vi "Set Button Complete.vi"(0 "Button in":refnum<class "Button.lvclass">, 1 "On Picture":picture, 2 "Disabled Picture":picture, 5 "Type":T1, 7 "State":T2, 9 "Off Picture":picture, 11 "error in (no error)":errorcluster, 12 "Hover Picture":picture, 13 "Button Size":i32) -> (4 "Button out":refnum<class "Button.lvclass">, 15 "error out":errorcluster)   [LabVIEW 2012, in "Button.lvclass"]
uses:
  Button.lvclass
  Type Defs/Button Status.ctl
  Type Defs/Button Type.ctl
  Button.lvclass/Button.ctl
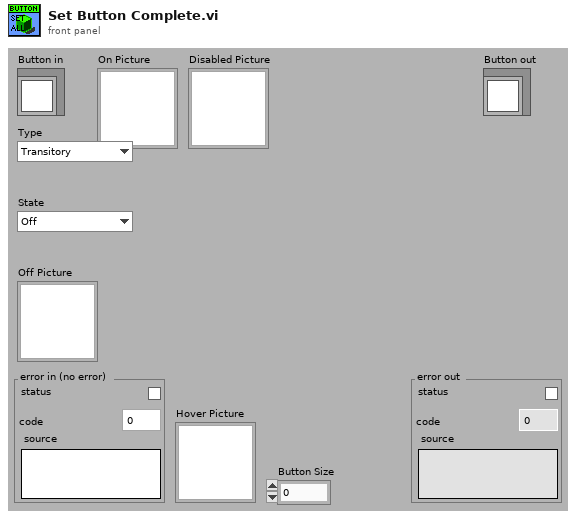
[diagram p1: front panel]
types:
  T1 = typedef "Button.lvclass/Button Type.ctl" = enum16{"Transitory", "Latching"}
  T2 = typedef "Button.lvclass/Button Status.ctl" = enum16{"Off", "Hover", "On", "Disabled"}
  T3 = typedef "imagedata.ctl" = cluster{"image type":i32, "image depth":i32, "image":u8[], "mask":u8[], "colors":u32[], "Rectangle":cluster{"left":i16, "top":i16, "right":i16, "bottom":i16}}
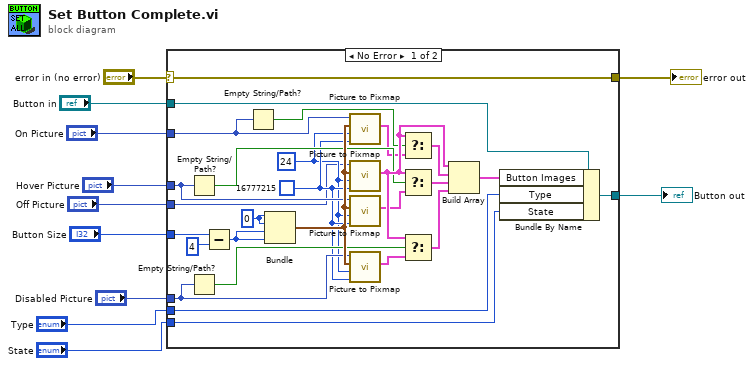
[diagram p0: block diagram]
diagram:
  n1 = case shown="No Error" "error in (no error)" {
    selector: "error in (no error)" -> [w12 w39]
    tunnel: "Button Size" -> [w36 _]
    tunnel: "Disabled Picture" -> [w22 _]
    tunnel: "Hover Picture" -> [w21 _]
    tunnel: "On Picture" -> [w18 _]
    tunnel: "Off Picture" -> [w17 _]
    tunnel: "State" -> [w16 _]
    tunnel: "Type" -> [w15 _]
    tunnel: [w14 w40] -> w4
    tunnel: "Button in" -> [w13 w40]
    tunnel: [w12 w39] -> w1
    frame No Error {
      w34 = 0
      w20 = u32 16777215 ("Background Color")
      w19 = 24 ("depth")
      n2 = Empty String/Path?(string/path=w21) -> (empty?=w25:bool)
      n3 = Empty String/Path?(string/path=w22) -> (empty?=w28:bool)
      n4 = Subtract(x=w36, y=4 ("x")) -> (x-y=w35:i32)
      n5 = Empty String/Path?(string/path=w18) -> (empty?=w23:bool)
      n6 = Bundle(w34, w34, w35, w35) -> (w33:cluster{i32, i32, i32, i32})  [unwired: 1 out]
      n7 = call <vilib>:"Picture to Pixmap.vi"("Background Color"=w20, "depth"=w19, "rect"=w33, "picture"=w18) -> ("image data"=w24:T3)  [unwired: 7 out]
      n8 = call <vilib>:"Picture to Pixmap.vi"("Background Color"=w20, "depth"=w19, "rect"=w33, "picture"=w17) -> ("image data"=w29:T3)  [unwired: 7 out]
      n9 = call <vilib>:"Picture to Pixmap.vi"("Background Color"=w20, "depth"=w19, "rect"=w33, "picture"=w21) -> ("image data"=w26:T3)  [unwired: 7 out]
      n10 = call <vilib>:"Picture to Pixmap.vi"("Background Color"=w20, "depth"=w19, "rect"=w33, "picture"=w22) -> ("image data"=w27:T3)  [unwired: 7 out]
      n11 = Select(t=w29, s=w23, f=w24) -> (s? t:f=w30:T3)
      n12 = Select(t=w29, s=w25, f=w26) -> (s? t:f=w31:T3)
      n13 = Select(t=w29, s=w28, f=w27) -> (s? t:f=w32:T3)
      n14 = Build Array(w29, w30, w31, w32) -> (w38:T3[])
      n15 = Bundle By Name(cluster=w13, "Button Images"=w38, "Type"=w15, "State"=w16) -> (w14:refnum<class "Button.lvclass">)
    }
    frame Error {
    }
  }
  "Button out" <- w4
  "error out" <- w1
